vi "SelectConfig.vi"(8 "error in":errorcluster) -> (0 "error constant":errorcluster, 1 "Cancel":bool, 2 "Config":string)   [LabVIEW 2024, in "Launcher_DTU.lvlib"]
uses:
  Launcher_DTU.lvlib
  Controls/Launch_Enum.ctl
panel:
  in  "Stop":bool
  in  "OK":bool
  in  "Configurations":u16(ring) items=["DTU_EOL", "DTU_EOL_2", "DTU_FCT"]
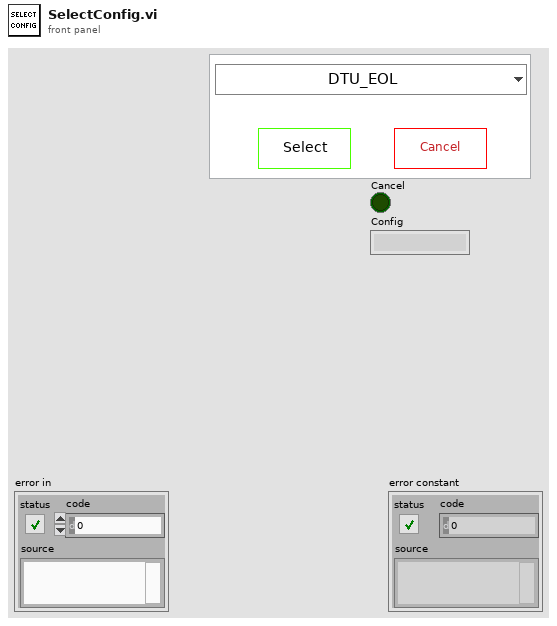
[diagram p1: front panel]
types:
  T1 = typedef "Launcher_DTU.lvlib/Launch_Enum.ctl" = enum16{"Init", "Poll", "LaunchScreen", "Exit"}
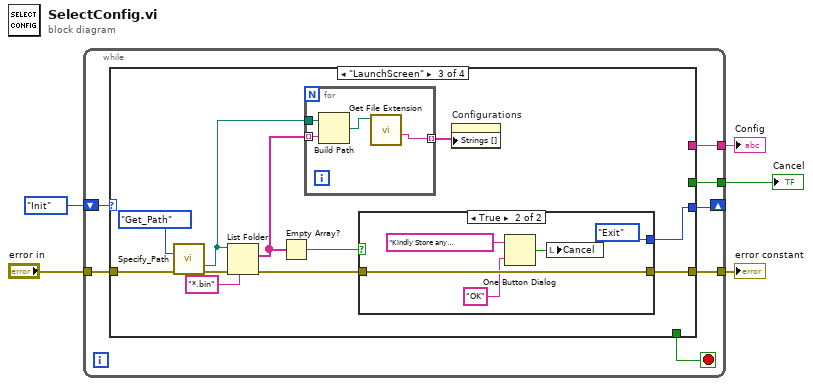
[diagram p0: block diagram]
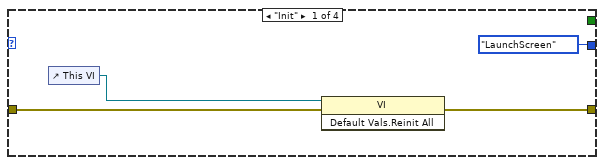
[diagram p2: hidden frame]
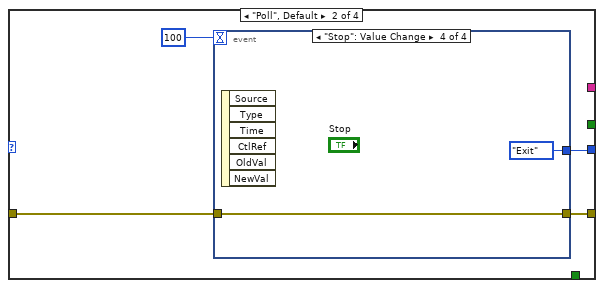
[diagram p3: hidden frame]
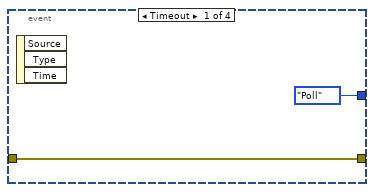
[diagram p4: hidden frame]
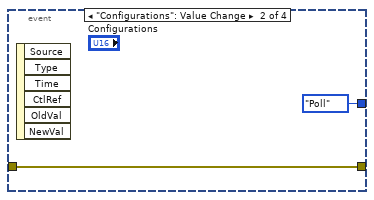
[diagram p5: hidden frame]
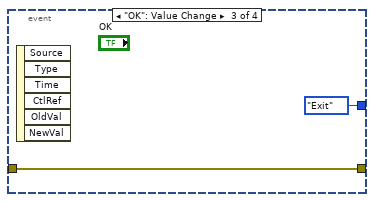
[diagram p6: hidden frame]
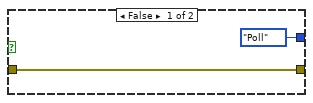
[diagram p7: hidden frame]
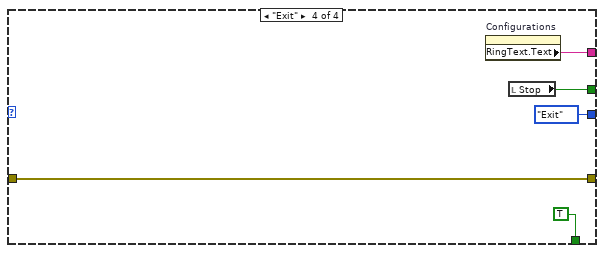
[diagram p8: hidden frame]
diagram:
  n1 = while {
    shift-right: [w11] -> _
    shift-left: Launch_Enum."Init" -> [w12]
    tunnel: "error in" -> [w10]
    tunnel: [w9] -> w3
    tunnel: [w7] -> w2
    tunnel: [w6] -> w1
    stop <- w8 stop-if-true
    n2 = case shown="\"LaunchScreen\"" w12 {
      tunnel: [Launch_Enum."LaunchScreen" w19 w32 Launch_Enum."Exit"] -> w11
      tunnel: w10 -> [w15 w18 w39 w54]
      tunnel: [w14 w17 w34 w54] -> w9
      tunnel: [_ _ _ TRUE] -> w8
      tunnel: [_ _ _ w52] -> w7
      tunnel: [_ _ _ w51] -> w6
      frame "Init" {
        n3 = control-ref of="This VI"() -> (w13:refnum<vi>)
        n4 = invoke class="VI" method="Default Vals.Reinit All"(reference=w13, error in=w15) -> (error out=w14:errorcluster)  [unwired: 1 in, 2 out]
      }
      frame "Poll", Default {
        n5 = event shown="[3] \"Stop\": Value Change" {
          selector: _ -> [_ _ _ _]
          dyn-events: _ -> [_ _ _ _]
          timeout: 100 -> [_ _ _ _]
          tunnel: [Launch_Enum."Poll" Launch_Enum."Poll" Launch_Enum."Exit" Launch_Enum."Exit"] -> w19
          tunnel: w18 -> [w21 w23 w25 w27]
          tunnel: [w21 w23 w25 w27] -> w17
          event Timeout {
            n6 = event-data() -> ()  [unwired: 1 in, 3 out]
          }
          event "Configurations": Value Change {
            n7 = event-data() -> ()  [unwired: 1 in, 6 out]
          }
          event "OK": Value Change {
            n8 = event-data() -> ()  [unwired: 1 in, 6 out]
          }
          event "Stop": Value Change {
            n9 = event-data() -> ()  [unwired: 1 in, 6 out]
          }
        }
      }
      frame "LaunchScreen" {
        n10 = call "Specify_Path.vi"("Path_Enum"=enum16{"Find_Path", "Get_Path"}."Get_Path", "error in (no error)"=w39) -> ("Settings"=w31:path, "error out"=w38:errorcluster)  [unwired: 6 in, 6 out]
        n11 = List Folder(path=w31, pattern="*.bin", error in=w38) -> (filenames=w30:string[], error out=w35:errorcluster)  [unwired: 1 in, 2 out]
        n12 = Empty Array?(array=w30) -> (empty?=w33:bool)
        n13 = for {
          tunnel: w31 -> [w42]
          tunnel: w30 -> [w41] mode=indexing
          tunnel: [w40] -> w29 mode=indexing
          n14 = Build Path(base path=w42, name or relative path=w41) -> (appended path=w43:path)
          n15 = call <vilib>:"Get File Extension.vi"("file"=w43) -> ("filename without extension"=w40:string)  [unwired: 6 in, 4 out]
        }
        n16 = case shown="True" w33 {
          tunnel: w35 -> [w45 w50]
          tunnel: [w45 w50] -> w34
          tunnel: [Launch_Enum."Poll" Launch_Enum."Exit"] -> w32
          frame False {
          }
          frame True {
            n17 = One Button Dialog(message="Kindly Store any Configurations from settings", button name ("OK")="OK") -> (true=w47:bool)
            n18 = local write "Cancel"(w47) -> ()
          }
        }
        n19 = property on="Configurations" class="Ring (strict)"("Strings []"=w29) -> ()  [unwired: 2 in, 2 out]
      }
      frame "Exit" {
        n20 = property on="Configurations" class="Ring (strict)"() -> ("RingText.Text"=w51:string)  [unwired: 2 in, 2 out]
        n21 = local read "Stop"() -> (w52:bool)
      }
    }
  }
  "error constant" <- w3
  "Cancel" <- w2
  "Config" <- w1
